vi "Modify Waveform in List.vi"(7 "Waveform List Ctl Ref":refnum<vi>, 8 "error in (no error)":errorcluster, 11 "Canvas Wfm Array In":waveform(dbl)[](array[waveform])) -> (0 "error out":errorcluster, 3 "Canvas Wfm Array Out":waveform(dbl)[](array[waveform]))   [LabVIEW 2025, in "TDMS Waveform Creator UI.lvlib"]
uses:
  TDMS Waveform Creator UI.lvlib
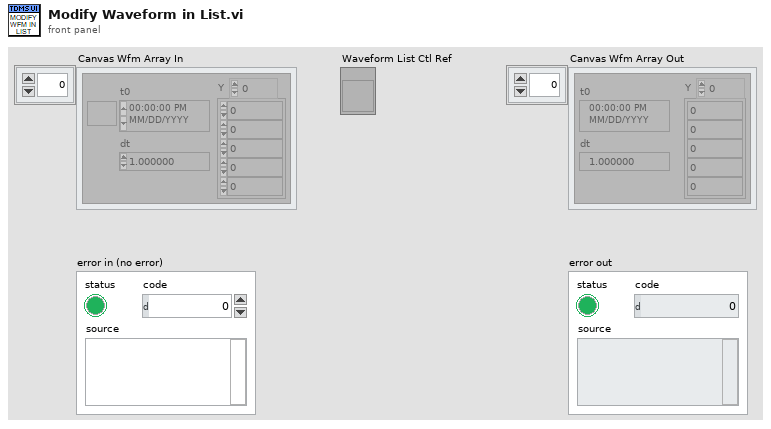
[diagram p1: front panel]
types:
  T1 = cluster{"File Path":string, "Sample Rate (Hz)":dbl, "Read From":i32, "Pre Delay (s)":dbl, "Post Delay (s)":dbl, "Scale":dbl}
  T2 = cluster{"Waveform Type":i32, "Sample Rate (Hz)":dbl, "Frequency (Hz)":dbl, "Amplitude":dbl, "Number of Cycles":u32, "Ramp Start":dbl, "Ramp Stop":dbl, "Length (s)":dbl, "DC Value":dbl, "Duration (s)":dbl, "Pre Delay (s)":dbl, "Post Delay (s)":dbl}
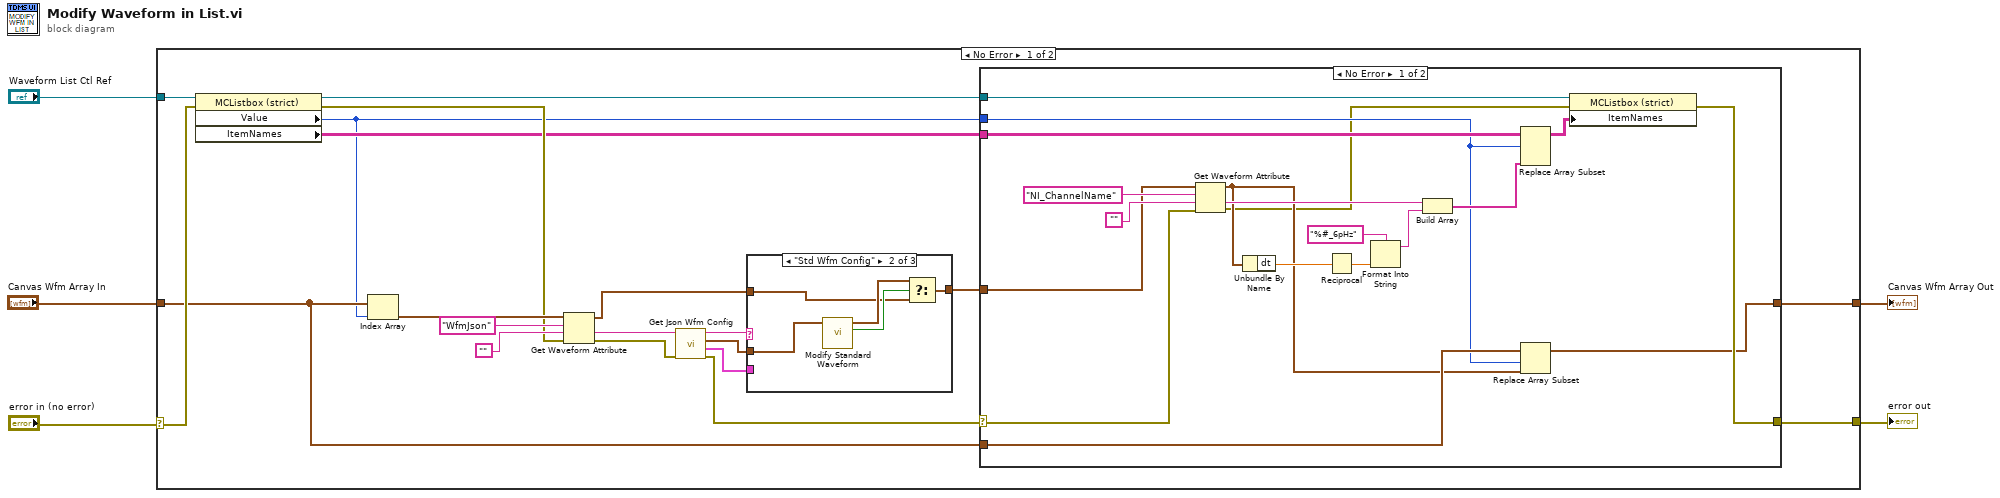
[diagram p0: block diagram]
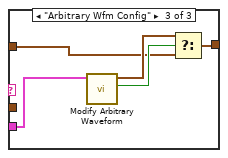
[diagram p4: hidden frame]
diagram:
  n1 = case shown="No Error" "error in (no error)" {
    selector: "error in (no error)" -> [w23 w59]
    tunnel: "Waveform List Ctl Ref" -> [w25 _]
    tunnel: "Canvas Wfm Array In" -> [w8 w58]
    tunnel: [w6 w58] -> w2
    tunnel: [w22 w59] -> w1
    frame No Error {
      n2 = property class="MCListbox (strict)"(reference=w25, error in=w23) -> (reference out=w24:refnum<vi>, error out=w18:errorcluster, "Value"=w7:i32, "ItemNames"=w9:string[][])
      n3 = Index Array(array=w8, index=w7) -> (element=w19:waveform(dbl))
      n4 = Get Waveform Attribute(4:w18, 5:"", 6:"WfmJson" ("name"), 7:w19) -> (0:w16:errorcluster, 1:w17:string, 3:w12:waveform(dbl))  [unwired: 1 out]
      n5 = call "Get Json Wfm Config.vi"("error in"=w16, "Json String"=w17) -> ("error out"=w10:errorcluster, "Arbitrary Wfm Config"=w13:T1, "Std Wfm Config"=w14:T2, "Type"=w15:string)  [unwired: 6 in]
      n6 = case shown="\"Std Wfm Config\"" w15 {
        tunnel: w14 -> [_ w52 _]
        tunnel: w13 -> [_ _ w53]
        tunnel: w12 -> [w47 w49 w55]
        tunnel: [w47 w48 w54] -> w11
        frame Default {
        }
        frame "Std Wfm Config" {
          n7 = call "Modify Standard Waveform.vi"("Standard Wfm Config"=w52) -> ("Waveform Modified?"=w51:bool, "Modified Waveform"=w50:waveform(dbl))  [unwired: 9 in]
          n8 = Select(t=w50, s=w51, f=w49) -> (s? t:f=w48:waveform(dbl))
        }
        frame "Arbitrary Wfm Config" {
          n9 = call "Modify Arbitrary Waveform.vi"("Arbitrary Wfm Config"=w53) -> ("Waveform Modified?"=w57:bool, "Modified Waveform"=w56:waveform(dbl))  [unwired: 9 in]
          n10 = Select(t=w56, s=w57, f=w55) -> (s? t:f=w54:waveform(dbl))
        }
      }
      n11 = case shown="No Error" w10 {
        selector: w10 -> [w34 w45]
        tunnel: w24 -> [w37 _]
        tunnel: [w36 w45] -> w22
        tunnel: w11 -> [w35 _]
        tunnel: w9 -> [w33 _]
        tunnel: w8 -> [w30 w46]
        tunnel: w7 -> [w28 _]
        tunnel: [w27 w46] -> w6
        frame No Error {
          n12 = Get Waveform Attribute(4:w34, 5:"", 6:"NI_ChannelName" ("name"), 7:w35) -> (0:w26:errorcluster, 1:w39:string, 3:w29:waveform(dbl))  [unwired: 1 out]
          n13 = Unbundle By Name(w29) -> ("dt"=w42:dbl)
          n14 = Reciprocal(x=w42) -> (1/x=w41:dbl)
          n15 = Format Into String(format string="%#_6pHz", w41) -> (resulting string=w38:string)  [unwired: 2 in, 1 out]
          n16 = Build Array(w39, w38) -> (w32:string[])
          n17 = Replace Array Subset(array=w33, new element=w32, index (row)=w28) -> (w31:string[][])  [unwired: 1 in]
          n18 = Replace Array Subset(array=w30, new element=w29, index=w28) -> (w27:waveform(dbl)[])
          n19 = property class="MCListbox (strict)"(reference=w37, error in=w26, "ItemNames"=w31) -> (error out=w36:errorcluster)  [unwired: 1 out]
        }
        frame Error {
        }
      }
    }
    frame Error {
    }
  }
  "error out" <- w1
  "Canvas Wfm Array Out" <- w2
